vi "Begin.vi"(8 "error in":errorcluster) -> (0 "error out":errorcluster)   [LabVIEW 2023]
doc: "Called before other user functions, this VI can be used to open I/O refnums, load in file data, and do general program initialization. Notice that the <B>error out</B> terminal is simply used for data flow. Wiring it to other structures or subVIs ensures that this VI runs first."
uses:
  <vilib>/Rock Robotics/WPI/DriverStation/WPI_DriverStationRobotMode2.ctl
  <vilib>/Rock Robotics/WPI/Joystick/WPI_JoystickDeviceEnum.ctl
  <vilib>/Rock Robotics/WPI/SafetyOutput/WPI_SafetyOutputConfigMenu.ctl
  <vilib>/Rock Robotics/WPI/ThirdParty/REV Robotics/REVLib/Typedef/Spark MAX Idle Mode.ctl
  Robot Global Data.vi
  <vilib>/Rock Robotics/Network Tables/NT Write String Array.vi
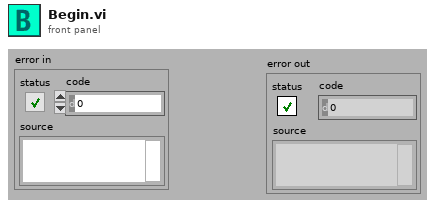
[diagram p1: front panel]
types:
  T1 = typedef "Spark MAX Idle Mode.ctl" = enum16{"Coast", "Brake"}
  T2 = typedef "WPI_SafetyOutputConfigMenu.ctl" = enum16{"Enable", "Disable"}
  T3 = typedef "WPI_JoystickDeviceEnum.ctl" = enum16{"USB 0", "USB 1", "USB 2", "USB 3", "USB 4", "USB 5"}
  T4 = typedef "WPI_DriverStationRobotMode2.ctl" = enum16{"Autonomous Disabled", "Autonomous Enabled", "Teleop Disabled", "Teleop Enabled", "Disconnected", "Finish", "Test Disabled", "Test Enabled", "Emergency Stopped"}
  T5 = typedef "WPI_MotorControlDeviceRef.ctl" = cluster{"DeviceStatus":errorcluster, "Type":T6, "PWM":cluster{"PWM Channel":T7, "DeadBand":T8}, "CAN":cluster{"Device Number":u8, "SetOutput VI Ref":variant, "GetOutput VI Ref":variant, "Enable VI Ref":variant, "Disable VI Ref":variant, "Data":variant}, "Invert":bool, "DIO PWM":cluster{"PWM \"Enable\" Channel":T7, "DIOChannel":T9, "PWM Rate":dbl}}
  T6 = typedef "WPI_MotorControlType.ctl" = enum16{"PWM", "CAN", "DIO PWM"}
  T7 = typedef "FPGA_DIOPWMChannel.ctl" = enum8{"PWM 0", "PWM 1", "PWM 2", "PWM 3", "PWM 4", "PWM 5", "PWM 6", "PWM 7", "PWM 8", "PWM 9", "PWM MXP 0", "PWM MXP 1", "PWM MXP 2", "PWM MXP 3", "PWM MXP 4", "PWM MXP 5", "PWM MXP 6", "PWM MXP 7", "PWM MXP 8", "PWM MXP 9", "Invalid"}
  T8 = typedef "WPI_PWMDeadband.ctl" = cluster{"Name":string, "maxPositivePwm":i32, "minPositivePwm":i32, "centerPwm":i32, "maxNegativePwm":i32, "minNegativePwm":i32, "angularRange":u16}
  T9 = typedef "FPGA_DIOChannel.ctl" = enum8{"DIO 0", "DIO 1", "DIO 2", "DIO 3", "DIO 4", "DIO 5", "DIO 6", "DIO 7", "DIO 8", "DIO 9", "DIO MXP 0", "DIO MXP 1", "DIO MXP 2", "DIO MXP 3", "DIO MXP 4", "DIO MXP 5", "DIO MXP 6", "DIO MXP 7", "DIO MXP 8", "DIO MXP 9", "DIO MXP 10", "DIO MXP 11", "DIO MXP 12", "DIO MXP 13", "DIO MXP 14", "DIO MXP 15", "SPI Port CS1", "SPI Port CS2", "SPI Port CS3", "SPI Port MISO", "SPI Port MOSI", "Invalid"}
  T10 = typedef "WPI_JoystickDevRef.ctl" = cluster{"Device":T3}
  T11 = typedef "ADIS16470 Device Reference.ctl" = cluster{"DevStatus":errorcluster, "Hardware Config":T12, "Calibration Complete":refnum<notifier>, "Status Reference":refnum<data-value>, "Data Reference":refnum<data-value>, "Sychronous Process VI":T15, "Cmd FIFO":refnum<k33>, "Source":T16, "Data FIFO":refnum<k33>, "Calibration Time (ms)":u32, "Data Reference":refnum<data-value>}
  T12 = typedef "ADIS16470 Hardware Configuration.ctl" = cluster{"SPI Clock Rate (Hz)":dbl, "IMU SPI Mode (3)":T13, "IMU Reset Pin":T9, "IMU SPI Bus":T14, "IMU Data Ready Pin":T9, "Stall Config":cluster{"Pow2BytesPerRead":u8, "StallTicks":u16, "CsToSclkTicks":u8}}
  T13 = typedef "WPI_SPIMode.ctl" = enum16{"Mode 0 (Clk Idle Low,Sample on Leading)", "Mode 1 (Clk Idle Low,Sample on Trailing)", "Mode 2 (Clk Idle High,Sample on Leading)", "Mode 3 (Clk Idle High,Sample on Trailing)"}
  T14 = typedef "spi_bus.ctl" = enum16{"SPI On-Board, CS0", "SPI On-Board, CS1", "SPI On-Board, CS2", "SPI On-Board, CS3", "SPI MXP", "Invalid"}
  T15 = typedef "ADIS16470 Process.ctl" = refnum<vi>
  T16 = typedef "FPGA_CounterEncoderSourceConvertionLVSourceType.ctl" = cluster{"DevStatus":errorcluster, "AnalogTriggerMode?":bool, "DigitalMode":cluster{"DIO Channel":T17}, "AnalogTriggerMode":cluster{"AnalogTriggerIndex":T18, "OutputType":T19}}
  T17 = typedef "FPGA_DIODigitalSourceChannel.ctl" = enum8{"DIO 0", "DIO 1", "DIO 2", "DIO 3", "DIO 4", "DIO 5", "DIO 6", "DIO 7", "DIO 8", "DIO 9", "DIO MXP 0", "DIO MXP 1", "DIO MXP 2", "DIO MXP 3", "DIO MXP 4", "DIO MXP 5", "DIO MXP 6", "DIO MXP 7", "DIO MXP 8", "DIO MXP 9", "DIO MXP 10", "DIO MXP 11", "DIO MXP 12", "DIO MXP 13", "DIO MXP 14", "DIO MXP 15", "SPI Port CS1", "SPI Port CS2", "SPI Port CS3", "SPI Port MISO", "SPI Port MOSI", "Disabled"}
  T18 = typedef "FPGA_AnalogTriggerIndex.ctl" = enum8{"Trig 0", "Trig 1", "Trig 2", "Trig 3", "Trig 4", "Trig 5", "Trig 6", "Trig 7", "Invalid"}
  T19 = typedef "FPGA_AnalogTriggerOutType.ctl" = enum16{"InWindow", "TriggerState", "Rising", "Falling"}
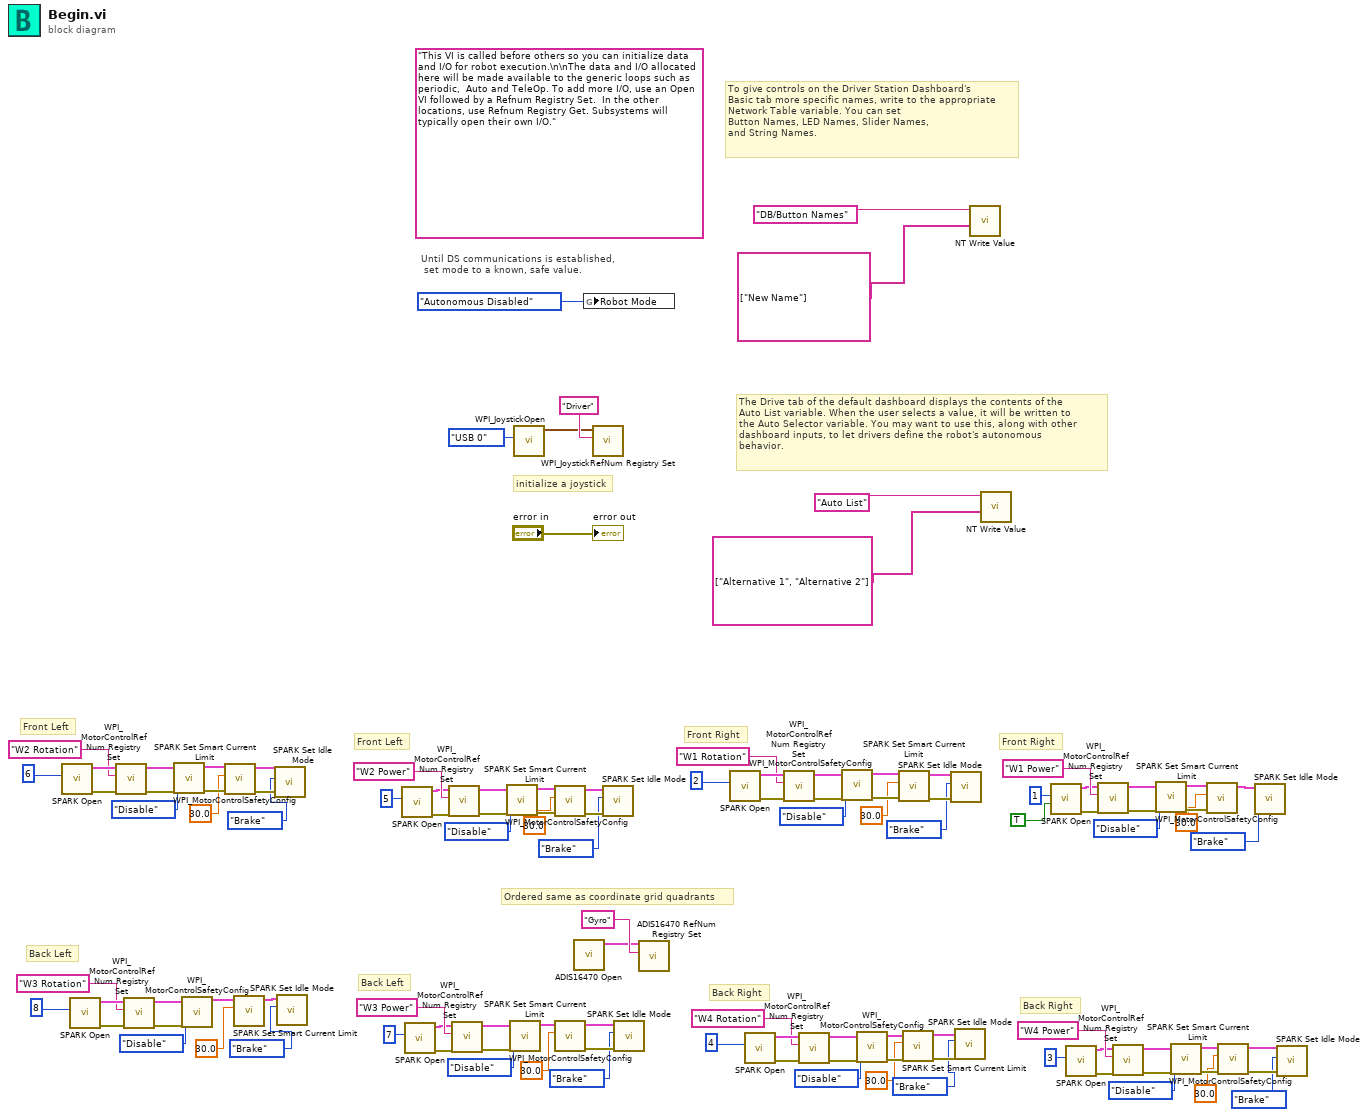
[diagram p0: block diagram]
diagram:
  (unwired) "This VI is called before others so you can initialize data and I/O for robot execution.\n\nThe data and I/O allocated here will be made available to the generic loops such as periodic,  Auto and TeleOp. To add more I/O, use an Open VI followed by a Refnum Registry Set.  In the other locations, use Refnum Registry Get. Subsystems will typically open their own I/O."
  # "Ordered same as coordinate grid quadrants"
  # "Back Right"
  # "Back Right"
  # "Back Left"
  # "Back Left"
  # "Front Left"
  # "Front Left"
  # "Front Right"
  # "Front Right"
  # "The Drive tab of the default dashboard displays the contents of the\nAuto List variable. When the user selects a value, it will be written to\nthe Auto Selector variable. You may want to use this, along with other\ndashboard inputs, to let drivers define the robot's autonomous\nbehavior."
  # "To give controls on the Driver Station Dashboard's\nBasic tab more specific names, write to the appropriate\nNetwork Table variable. You can set\nButton Names, LED Names, Slider Names,\nand String Names."
  # "initialize a joystick"
  # "Until DS communications is established,\n set mode to a known, safe value."
  n1 = call <vilib>:"SPARK Open.vi"("Device Number"=u8 6) -> ("error out"=w90:errorcluster, "MotorControlDeviceRef"=w89:T5)  [unwired: 9 in]
  n2 = call <vilib>:"SPARK Open.vi"("Device Number"=u8 8) -> ("error out"=w78:errorcluster, "MotorControlDeviceRef"=w77:T5)  [unwired: 9 in]
  n3 = call <vilib>:"WPI_MotorControlRefNum Registry Set.vi"("error in (no error)"=w90, "refnum name"="W2 Rotation", "MotorControlDevRef"=w89) -> ("error out"=w88:errorcluster, "MotorControlDevRef"=w26:T5)  [unwired: 7 in]
  n4 = call <vilib>:"WPI_MotorControlRefNum Registry Set.vi"("error in (no error)"=w78, "refnum name"="W3 Rotation", "MotorControlDevRef"=w77) -> ("error out"=w76:errorcluster, "MotorControlDevRef"=w75:T5)  [unwired: 7 in]
  n5 = call <vilib>:"WPI_MotorControlSafetyConfig.vi"("error in (no error)"=w88, "mode"=WPI_SafetyOutputConfigMenu."Disable", "MotorControlDevRef"=w26) -> ("error out"=w29:errorcluster, "MotorControlDevRef"=w28:T5)  [unwired: 7 in]
  n6 = call <vilib>:"WPI_MotorControlSafetyConfig.vi"("error in (no error)"=w76, "mode"=WPI_SafetyOutputConfigMenu."Disable", "MotorControlDevRef"=w75) -> ("MotorControlDevRef"=w48:T5)  [unwired: 7 in, 1 out]
  n7 = call <vilib>:"SPARK Set Smart Current Limit.vi"("error in (no error)"=w29, "Primay Current Limit (80A)"=30.0, "MotorControlDeviceRef in"=w28) -> ("error out"=w14:errorcluster, "MotorControlDeviceRef out"=w13:T5)  [unwired: 7 in]
  n8 = call <vilib>:"SPARK Set Smart Current Limit.vi"("Primay Current Limit (80A)"=30.0, "MotorControlDeviceRef in"=w48) -> ("MotorControlDeviceRef out"=w15:T5)  [unwired: 8 in, 1 out]
  n9 = call <vilib>:"SPARK Set Idle Mode.vi"("error in (no error)"=w14, "Idle Mode"=Spark_MAX_Idle_Mode."Brake", "MotorControlDeviceRef in"=w13) -> ()  [unwired: 7 in, 2 out]
  n10 = call <vilib>:"SPARK Set Idle Mode.vi"("Idle Mode"=Spark_MAX_Idle_Mode."Brake", "MotorControlDeviceRef in"=w15) -> ()  [unwired: 8 in, 2 out]
  n11 = call <vilib>:"SPARK Open.vi"("Device Number"=u8 5) -> ("error out"=w80:errorcluster, "MotorControlDeviceRef"=w81:T5)  [unwired: 9 in]
  n12 = call <vilib>:"SPARK Open.vi"("Device Number"=u8 7) -> ("error out"=w67:errorcluster, "MotorControlDeviceRef"=w68:T5)  [unwired: 9 in]
  n13 = call <vilib>:"WPI_MotorControlRefNum Registry Set.vi"("error in (no error)"=w80, "refnum name"="W2 Power", "MotorControlDevRef"=w81) -> ("error out"=w85:errorcluster, "MotorControlDevRef"=w84:T5)  [unwired: 7 in]
  n14 = call <vilib>:"WPI_MotorControlRefNum Registry Set.vi"("error in (no error)"=w67, "refnum name"="W3 Power", "MotorControlDevRef"=w68) -> ("error out"=w72:errorcluster, "MotorControlDevRef"=w71:T5)  [unwired: 7 in]
  n15 = call <vilib>:"WPI_MotorControlSafetyConfig.vi"("error in (no error)"=w85, "mode"=WPI_SafetyOutputConfigMenu."Disable", "MotorControlDevRef"=w84) -> ("error out"=w32:errorcluster, "MotorControlDevRef"=w31:T5)  [unwired: 7 in]
  n16 = call <vilib>:"WPI_MotorControlSafetyConfig.vi"("error in (no error)"=w72, "mode"=WPI_SafetyOutputConfigMenu."Disable", "MotorControlDevRef"=w71) -> ("MotorControlDevRef"=w46:T5)  [unwired: 7 in, 1 out]
  n17 = call <vilib>:"WPI_JoystickOpen.vi"("JoystickDevice"=WPI_JoystickDeviceEnum."USB 0") -> ("JoystickDevRef"=w110:T10)  [unwired: 10 in]
  n18 = call <vilib>:"SPARK Set Smart Current Limit.vi"("error in (no error)"=w32, "Primay Current Limit (80A)"=30.0, "MotorControlDeviceRef in"=w31) -> ("error out"=w18:errorcluster, "MotorControlDeviceRef out"=w17:T5)  [unwired: 7 in]
  n19 = call <vilib>:"SPARK Set Smart Current Limit.vi"("Primay Current Limit (80A)"=30.0, "MotorControlDeviceRef in"=w46) -> ("error out"=w20:errorcluster, "MotorControlDeviceRef out"=w19:T5)  [unwired: 8 in]
  n20 = call <vilib>:"ADIS16470 Open.vi"() -> ("ADIS16470DevRef"=w1:T11)  [unwired: 10 in, 1 out]
  n21 = global write "Robot Global Data.vi" "Robot Mode"(WPI_DriverStationRobotMode2."Autonomous Disabled" ("Robot Mode")) -> ()
  n22 = call <vilib>:"WPI_JoystickRefNum Registry Set.vi"("refnum name"="Driver", "JoystickDevRef"=w110) -> ()  [unwired: 8 in, 2 out]
  n23 = call <vilib>:"SPARK Set Idle Mode.vi"("error in (no error)"=w18, "Idle Mode"=Spark_MAX_Idle_Mode."Brake", "MotorControlDeviceRef in"=w17) -> ()  [unwired: 7 in, 2 out]
  n24 = call <vilib>:"SPARK Set Idle Mode.vi"("error in (no error)"=w20, "Idle Mode"=Spark_MAX_Idle_Mode."Brake", "MotorControlDeviceRef in"=w19) -> ()  [unwired: 7 in, 2 out]
  n25 = call <vilib>:"ADIS16470 RefNum Registry Set.vi"("refnum name"="Gyro", "ADIS16470DevRef in"=w1) -> ()  [unwired: 8 in, 2 out]
  n26 = call <vilib>:"SPARK Open.vi"("Device Number"=u8 2) -> ("error out"=w103:errorcluster, "MotorControlDeviceRef"=w102:T5)  [unwired: 9 in]
  n27 = call <vilib>:"SPARK Open.vi"("Device Number"=u8 4) -> ("error out"=w65:errorcluster, "MotorControlDeviceRef"=w64:T5)  [unwired: 9 in]
  n28 = call <vilib>:"WPI_MotorControlRefNum Registry Set.vi"("error in (no error)"=w103, "refnum name"="W1 Rotation", "MotorControlDevRef"=w102) -> ("error out"=w101:errorcluster, "MotorControlDevRef"=w100:T5)  [unwired: 7 in]
  n29 = call <vilib>:"WPI_MotorControlRefNum Registry Set.vi"("error in (no error)"=w65, "refnum name"="W4 Rotation", "MotorControlDevRef"=w64) -> ("error out"=w63:errorcluster, "MotorControlDevRef"=w62:T5)  [unwired: 7 in]
  n30 = call <vilib>:"WPI_MotorControlSafetyConfig.vi"("error in (no error)"=w101, "mode"=WPI_SafetyOutputConfigMenu."Disable", "MotorControlDevRef"=w100) -> ("error out"=w35:errorcluster, "MotorControlDevRef"=w34:T5)  [unwired: 7 in]
  n31 = call <vilib>:"WPI_MotorControlSafetyConfig.vi"("error in (no error)"=w63, "mode"=WPI_SafetyOutputConfigMenu."Disable", "MotorControlDevRef"=w62) -> ("error out"=w44:errorcluster, "MotorControlDevRef"=w43:T5)  [unwired: 7 in]
  n32 = call <vilib>:"SPARK Set Smart Current Limit.vi"("error in (no error)"=w35, "Primay Current Limit (80A)"=30.0, "MotorControlDeviceRef in"=w34) -> ("error out"=w10:errorcluster, "MotorControlDeviceRef out"=w9:T5)  [unwired: 7 in]
  n33 = call <vilib>:"SPARK Set Smart Current Limit.vi"("error in (no error)"=w44, "Primay Current Limit (80A)"=30.0, "MotorControlDeviceRef in"=w43) -> ("error out"=w8:errorcluster, "MotorControlDeviceRef out"=w7:T5)  [unwired: 7 in]
  n34 = call <vilib>:"SPARK Set Idle Mode.vi"("error in (no error)"=w10, "Idle Mode"=Spark_MAX_Idle_Mode."Brake", "MotorControlDeviceRef in"=w9) -> ()  [unwired: 7 in, 2 out]
  n35 = call <vilib>:"SPARK Set Idle Mode.vi"("error in (no error)"=w8, "Idle Mode"=Spark_MAX_Idle_Mode."Brake", "MotorControlDeviceRef in"=w7) -> ()  [unwired: 7 in, 2 out]
  n36 = call-poly <vilib>:"NT Write Value.vi"("value"=string[] ["New Name"] ("String Array"), "name"="DB/Button Names" ("Name")) -> ()  [unwired: 9 in, 1 out]
  n37 = call-poly <vilib>:"NT Write Value.vi"("value"=string[] ["Alternative 1", "Alternative 2"] ("String Array"), "name"="Auto List" ("Name")) -> ()  [unwired: 9 in, 1 out]
  n38 = call <vilib>:"SPARK Open.vi"("Invert"=TRUE, "Device Number"=u8 1) -> ("error out"=w92:errorcluster, "MotorControlDeviceRef"=w93:T5)  [unwired: 8 in]
  n39 = call <vilib>:"SPARK Open.vi"("Device Number"=u8 3) -> ("error out"=w54:errorcluster, "MotorControlDeviceRef"=w55:T5)  [unwired: 9 in]
  n40 = call <vilib>:"WPI_MotorControlRefNum Registry Set.vi"("error in (no error)"=w92, "refnum name"="W1 Power", "MotorControlDevRef"=w93) -> ("error out"=w97:errorcluster, "MotorControlDevRef"=w96:T5)  [unwired: 7 in]
  n41 = call <vilib>:"WPI_MotorControlRefNum Registry Set.vi"("error in (no error)"=w54, "refnum name"="W4 Power", "MotorControlDevRef"=w55) -> ("error out"=w59:errorcluster, "MotorControlDevRef"=w58:T5)  [unwired: 7 in]
  n42 = call <vilib>:"WPI_MotorControlSafetyConfig.vi"("error in (no error)"=w97, "mode"=WPI_SafetyOutputConfigMenu."Disable", "MotorControlDevRef"=w96) -> ("error out"=w38:errorcluster, "MotorControlDevRef"=w37:T5)  [unwired: 7 in]
  n43 = call <vilib>:"WPI_MotorControlSafetyConfig.vi"("error in (no error)"=w59, "mode"=WPI_SafetyOutputConfigMenu."Disable", "MotorControlDevRef"=w58) -> ("error out"=w41:errorcluster, "MotorControlDevRef"=w40:T5)  [unwired: 7 in]
  n44 = call <vilib>:"SPARK Set Smart Current Limit.vi"("error in (no error)"=w38, "Primay Current Limit (80A)"=30.0, "MotorControlDeviceRef in"=w37) -> ("MotorControlDeviceRef out"=w23:T5)  [unwired: 7 in, 1 out]
  n45 = call <vilib>:"SPARK Set Smart Current Limit.vi"("error in (no error)"=w41, "Primay Current Limit (80A)"=30.0, "MotorControlDeviceRef in"=w40) -> ("error out"=w22:errorcluster, "MotorControlDeviceRef out"=w21:T5)  [unwired: 7 in]
  n46 = call <vilib>:"SPARK Set Idle Mode.vi"("Idle Mode"=Spark_MAX_Idle_Mode."Brake", "MotorControlDeviceRef in"=w23) -> ()  [unwired: 8 in, 2 out]
  n47 = call <vilib>:"SPARK Set Idle Mode.vi"("error in (no error)"=w22, "Idle Mode"=Spark_MAX_Idle_Mode."Brake", "MotorControlDeviceRef in"=w21) -> ()  [unwired: 7 in, 2 out]
  "error out" <- "error in"
